vi "Global Has Mid Offset.vi"(0 "Has M Offset? in":bool, 3 "Set Data?":bool) -> (7 "Has M Offset? out":bool)   [LabVIEW 2019]
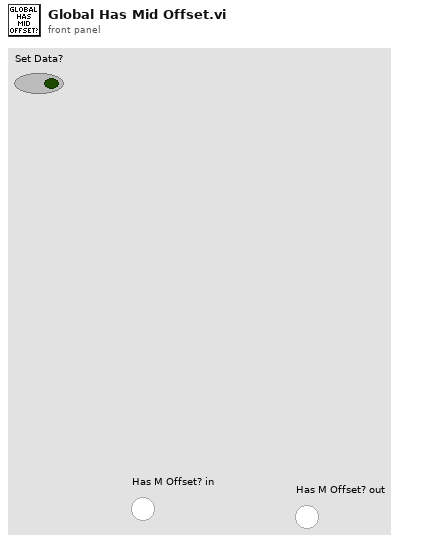
[diagram p1: front panel]
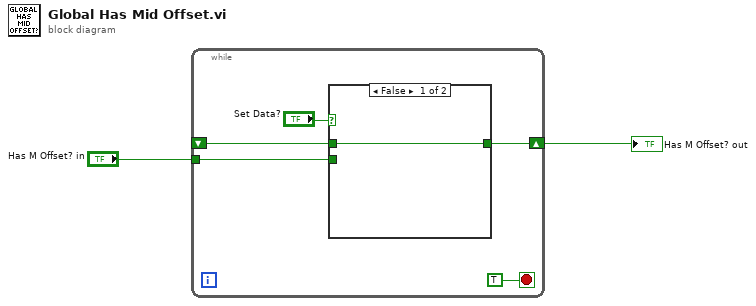
[diagram p0: block diagram]
diagram:
  n1 = while {
    shift-right: [w5] -> w2
    shift-left: _ -> [w4]
    tunnel: "Has M Offset? in" -> [w3]
    stop <- TRUE stop-if-true
    n2 = case shown="False" "Set Data?" {
      tunnel: [w8 w9] -> w5
      tunnel: w4 -> [w8 _]
      tunnel: w3 -> [_ w9]
      frame False {
      }
      frame True {
      }
    }
  }
  "Has M Offset? out" <- w2
